vi "DataCon.vi"() -> ()   [LabVIEW 2019]
uses:
  <vilib>/Utility/file.llb/Read Delimited Spreadsheet (string).vi
  <vilib>/Utility/file.llb/Write Delimited Spreadsheet (string).vi
panel:
  out "Total_Files":i32
  out "Output_File":path
  out "CSV_Files":path[](array[path])
  out "type":string
  out "All Files in Dir":path[](array[path])
  out "Processing_File":i32
  in  "Folder":path
  in  "error in (no error)":errorcluster
  out "all rows":string[][](array[string])
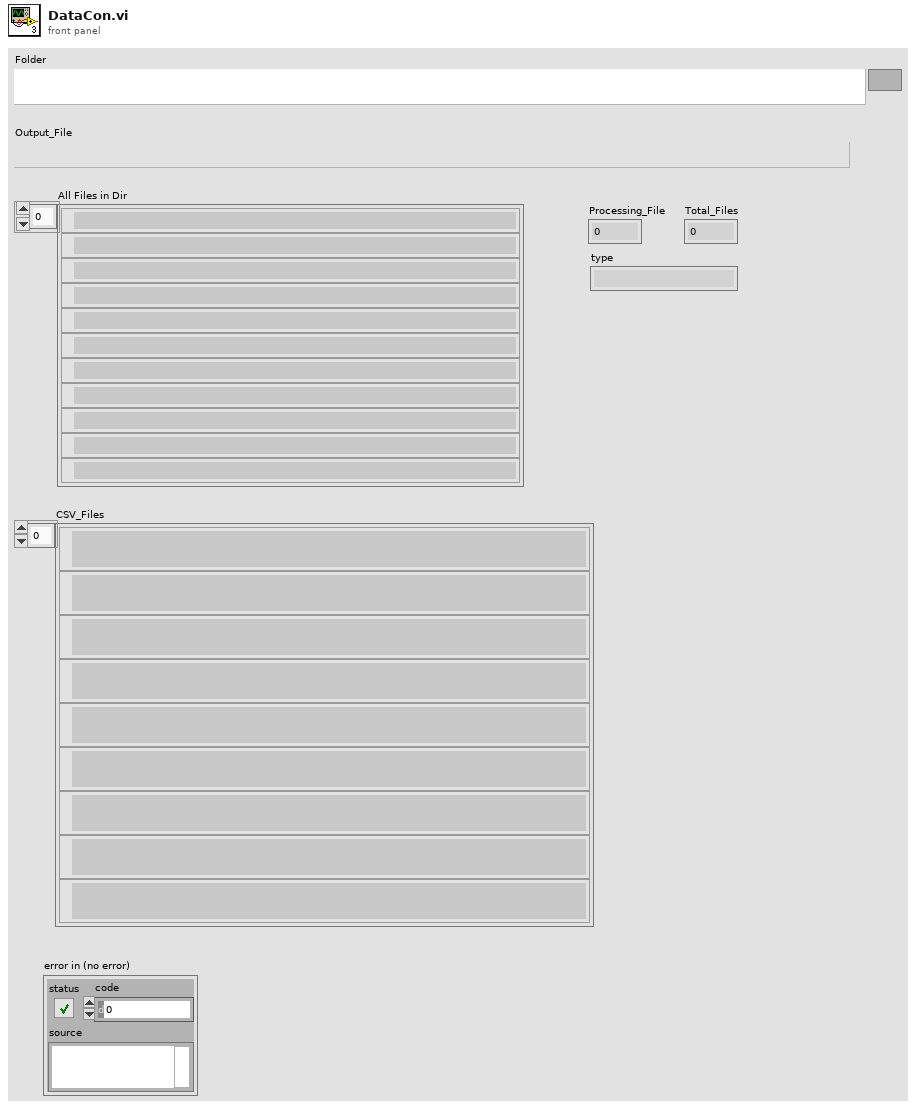
[diagram p1: front panel]
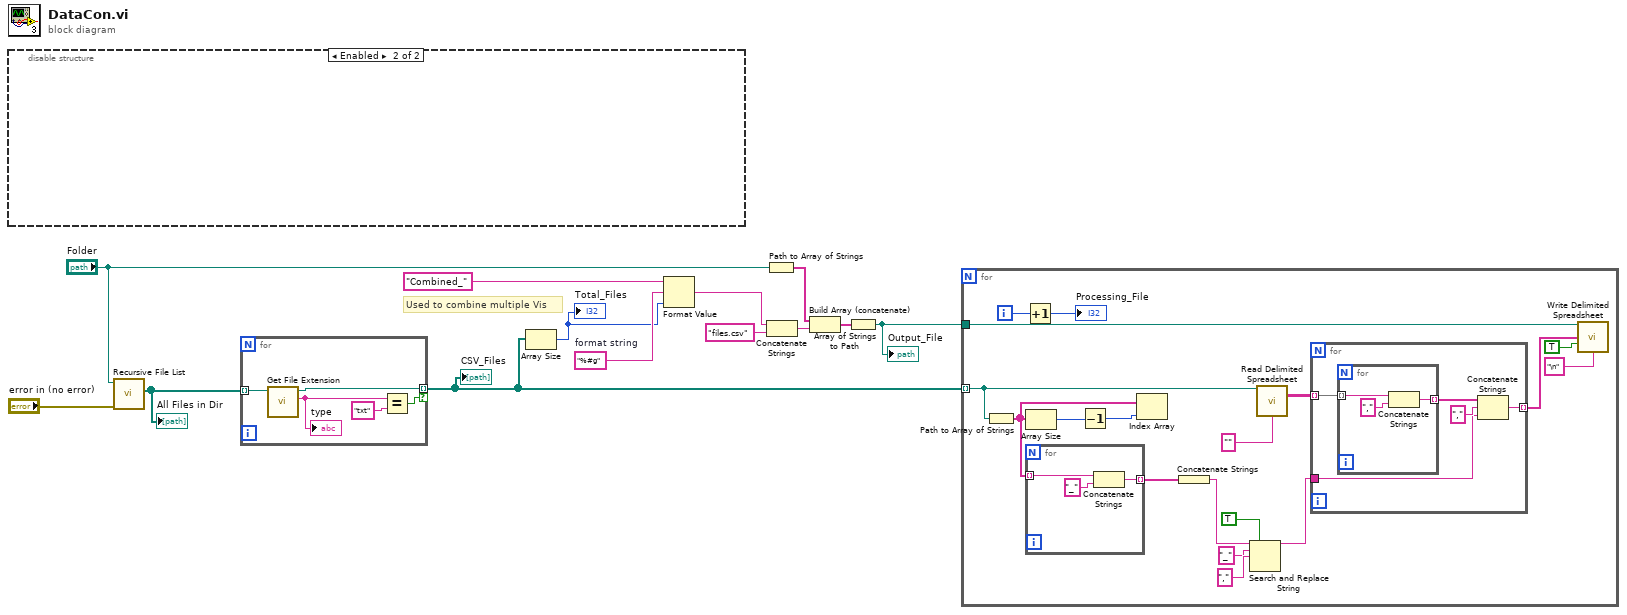
[diagram p0: block diagram]
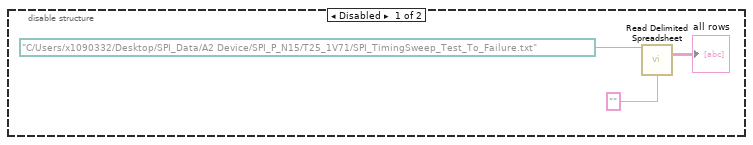
[diagram p2: hidden frame]
diagram:
  w4 = "%#g"  # format string
  # "Used to combine multiple Vis"
  n1 = disable-structure shown="Enabled" {
    frame Disabled {
      n2 = call-poly <vilib>:"Read Delimited Spreadsheet.vi"("file path (dialog if empty)"=path "C:/Users/x1090332/Desktop/SPI_Data/A2 Device/SPI_P_N15/T25_1V71/SPI_TimingSweep_Test_To_Failure.txt", "delimiter (\\t)"="" ("delimiter (\\t)")) -> ("all rows"=→"all rows":string[][])  [unwired: 8 in, 5 out]
    }
    frame Enabled {
    }
  }
  n3 = call <vilib>:"Recursive File List.vi"("error in (no error)"="error in (no error)", "Folder Path"="Folder") -> ("All Files in Dir"=w13:path[])  [unwired: 5 in, 4 out]
  "All Files in Dir" <- w13
  n4 = for {
    tunnel: w13 -> [w19] mode=indexing
    tunnel: [w18] -> w2 mode=indexing if=w17
    n5 = call <vilib>:"Get File Extension.vi"("file"=w19) -> ("lowercase file extension"=w21:string, "dup file"=w18:path)  [unwired: 6 in, 3 out]
    "type" <- w21
    n6 = Equal?(x=w21, y="txt") -> (x = y?=w17:bool)
  }
  "CSV_Files" <- w2
  n7 = Array Size(array=w2) -> (size(s)=w1:i32)
  "Total_Files" <- w1
  n8 = Format Value(string ("")="Combined_" ("y"), format string=w4, value (0)=w1) -> (output string=w6:string)
  n9 = Path to Array of Strings(0:"Folder") -> (2:w10:string[])  [unwired: 1 out]
  n10 = Concatenate Strings(w6, "files.csv" ("y")) -> (w7:string)
  n11 = Build Array (concatenate)(w10, w7) -> (w9:string[])
  n12 = Array of Strings to Path(0:w9) -> (2:w8:path)  [unwired: 1 in]
  "Output_File" <- w8
  n13 = for {
    tunnel: w2 -> [w31] mode=indexing
    tunnel: w8 -> [w27]
    i -> [w26]
    n14 = Path to Array of Strings(0:w31) -> (2:w25:string[])  [unwired: 1 out]
    n15 = Increment(x=w26) -> (x+1=→"Processing_File":i32)
    n16 = Array Size(array=w25) -> (size(s)=w30:i32)
    n17 = for {
      tunnel: w25 -> [w42] mode=indexing
      tunnel: [w40] -> w24 mode=indexing
      n18 = Concatenate Strings(w42, "_" ("string")) -> (w40:string)
    }
    n19 = Decrement(x=w30) -> (x-1=w29:i32)
    n20 = Index Array(array=w25, index=w29) -> ()  [unwired: 1 out]
    n21 = Concatenate Strings(w24) -> (w23:string)
    n22 = Search and Replace String(replace all?=TRUE ("replace all? (F)"), input string=w23, search string="_", replace string="," ("replace string (\"\")")) -> (result string=w34:string)  [unwired: 4 in, 3 out]
    n23 = call-poly <vilib>:"Read Delimited Spreadsheet.vi"("file path (dialog if empty)"=w31, "delimiter (\\t)"="" ("delimiter (\\t)")) -> ("all rows"=w39:string[][])  [unwired: 8 in, 5 out]
    n24 = for {
      tunnel: w39 -> [w44] mode=indexing
      tunnel: w34 -> [w46]
      tunnel: [w45] -> w36 mode=indexing
      n25 = for {
        tunnel: w44 -> [w50] mode=indexing
        tunnel: [w48] -> w43 mode=indexing
        n26 = Concatenate Strings(w50, "," ("delimiter (\\t)")) -> (w48:string)
      }
      n27 = Concatenate Strings(w43, "," ("delimiter (\\t)"), w46) -> (w45:string)
    }
    n28 = call-poly <vilib>:"Write Delimited Spreadsheet.vi"("file path (dialog if empty)"=w27, "1D data"=w36, "append to file? (new file:F)"=TRUE, "delimiter (\\t)"="\n" ("delimiter (\\t)")) -> ()  [unwired: 10 in, 2 out]
  }
